vi "Asylum_Driver_GetXYSetPoints.vi"(8 "error in (no error)":errorcluster, 11 "Application":refnum<k7>) -> (0 "error out":errorcluster, 1 "Y Setpoint":dbl, 2 "X Setpoint":dbl, 3 "Application":refnum<k7>)   [LabVIEW 2020]
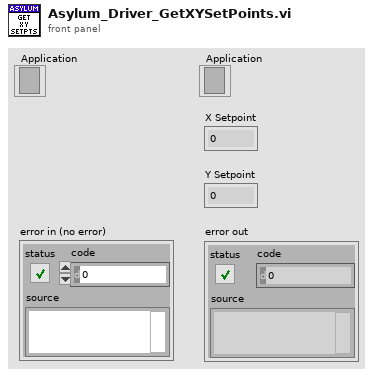
[diagram p1: front panel]
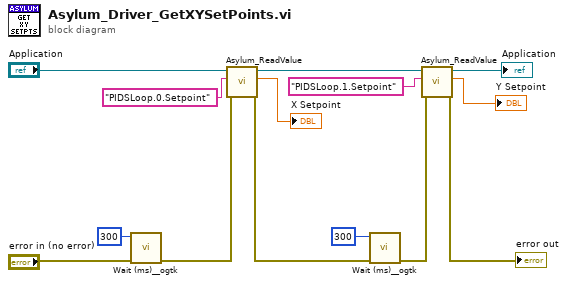
[diagram p0: block diagram]
diagram:
  n1 = call <userlib>:"Wait (ms)__ogtk.vi"("error in (no error)"="error in (no error)", "milliseconds to wait"=u32 300) -> ("error out"=w5:errorcluster)  [unwired: 8 in, 1 out]
  n2 = call <vilib>:"Asylum_ReadValue.vi"("error in (no error)"=w5, "Value"="PIDSLoop.0.Setpoint", "Application"="Application") -> ("error out"=w7:errorcluster, "Value"=→"X Setpoint":dbl, "Application"=w9:refnum<k7>)  [unwired: 6 in]
  n3 = call <userlib>:"Wait (ms)__ogtk.vi"("error in (no error)"=w7, "milliseconds to wait"=u32 300) -> ("error out"=w8:errorcluster)  [unwired: 8 in, 1 out]
  n4 = call <vilib>:"Asylum_ReadValue.vi"("error in (no error)"=w8, "Value"="PIDSLoop.1.Setpoint", "Application"=w9) -> ("error out"=→"error out":errorcluster, "Value"=→"Y Setpoint":dbl, "Application"=→"Application":refnum<k7>)  [unwired: 6 in]
